vi "TDMS Init_XNET.vi"(8 "error in (no error)":errorcluster, 9 "sbRIO?":bool=TRUE, 10 "group name":string, 11 "tdms file":refnum<k34>) -> (0 "error out":errorcluster, 3 "tdms file out":refnum<k34>)   [LabVIEW 2015]
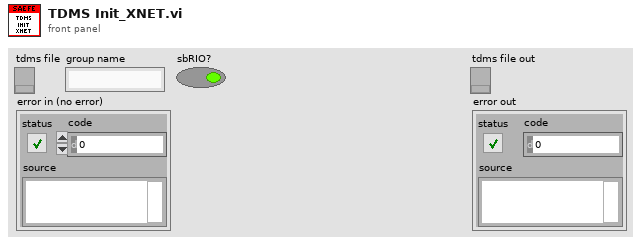
[diagram p1: front panel]
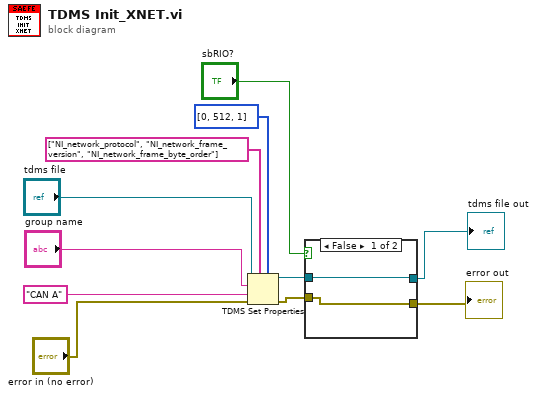
[diagram p0: block diagram]
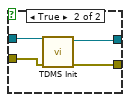
[diagram p2: hidden frame]
diagram:
  n1 = TDMS Set Properties(5:i32[] [0, 512, 1] ("property values"), 7:string[] ["NI_network_protocol", "NI_network_frame_version", "NI_network_frame_byte_order"] ("property names"), 8:"error in (no error)", 9:"CAN A" ("channel name"), 10:"group name", 11:"tdms file") -> (0:w4:errorcluster, 3:w5:refnum<k34>)  [unwired: 2 out]
  n2 = case shown="False" "sbRIO?" {
    tunnel: w5 -> [w13 w17]
    tunnel: w4 -> [w12 w16]
    tunnel: [w13 w15] -> w3
    tunnel: [w12 w14] -> w2
    frame False {
    }
    frame True {
      n3 = call "TDMS Init.vi"("error in (no error)"=w16, "tdms file"=w17) -> ("error out"=w14:errorcluster, "tdms file out"=w15:refnum<k34>)  [unwired: 8 in]
    }
  }
  "tdms file out" <- w3
  "error out" <- w2
